vi "Write Header.vi"(6 "Error In":errorcluster, 9 "File Refnum In":refnum<file>) -> (0 "Error Out":errorcluster, 3 "File Refnum Out":refnum<file>)   [LabVIEW 2014]
doc: "The VI auto-generates a string based on date and time and opens a file using the date time string as a file name. An array containing a sine and square wave is converted to a tab delimited string and written to the file. The file is then closed."
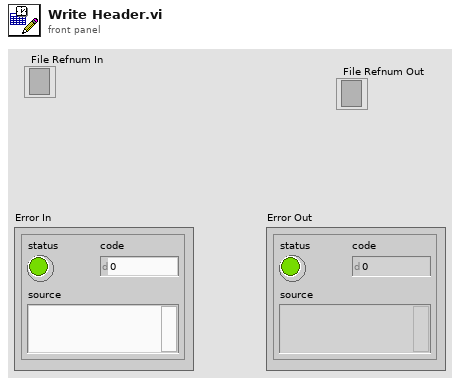
[diagram p1: front panel]
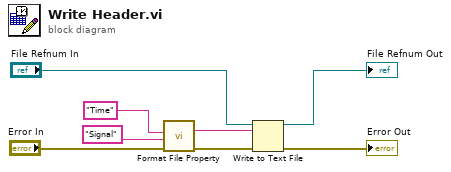
[diagram p0: block diagram]
diagram:
  n1 = call "Format File Property.vi"("Error In"="Error In", "File Property Value"="Signal", "File Property Name"="Time") -> ("Error Out"=w4:errorcluster, "String out"=w3:string)  [unwired: 7 in]
  n2 = Write to Text File(file (use dialog)="File Refnum In", text=w3, error in=w4) -> (refnum out=→"File Refnum Out":refnum<file>, error out=→"Error Out":errorcluster)  [unwired: 1 in, 1 out]
